vi "Generate Playlist XML String.vi"() -> ()   [LabVIEW 2011]
panel:
  out "XML String":string
  in  "Playlist":T1={"#attributes"={"Version"="1.0", "Creator"="LabVIEW"}, "Name"="Funky Grooves", "Song"=[{"Title"="Super Freak", "Artist"="Rick James"}, {"Title"="U Can't Touch This", "Artist"="MC Hammer"}, {"Title"="I Got You (I Feel Good)", "Artist"="James Brown"}, {"Title"="Get Down On It", "Artist"="Kool & The Gang"}]}
  # "Run this VI to generate a Playlist XML string (right) from the Playlist data structure (left)"
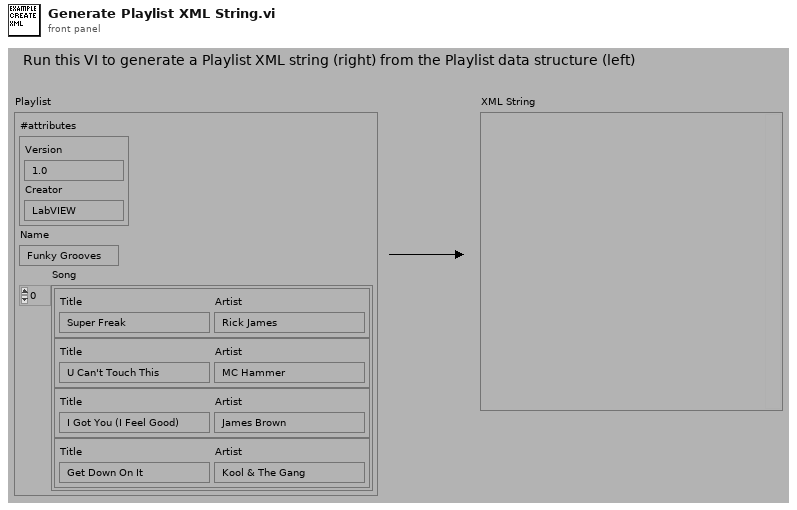
[diagram p1: front panel]
types:
  T1 = cluster{"#attributes":cluster{"Version":string, "Creator":string}, "Name":string, "Song":cluster{"Title":string, "Artist":string}[]}
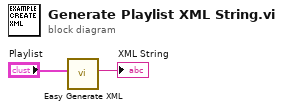
[diagram p0: block diagram]
diagram:
  n1 = call "Easy Generate XML.vi"("LabVIEW Data"="Playlist") -> ("XML String"=→"XML String":string)  [unwired: 9 in, 1 out]
